vi "splitter.vi"(3 "Npp_Frame":i32, 4 "Current":dbl[](array[numeric]), 5 "Voltage":dbl[](array[numeric])) -> (1 "Current Array":dbl[][](array[numeric]), 2 "Voltage Array":dbl[][](array[numeric]))   [LabVIEW 2018]
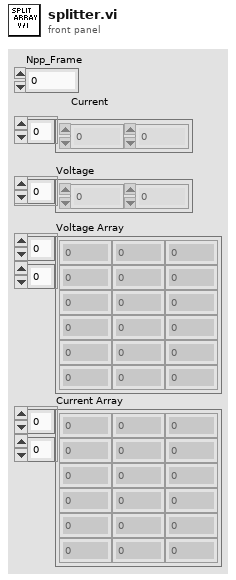
[diagram p1: front panel]
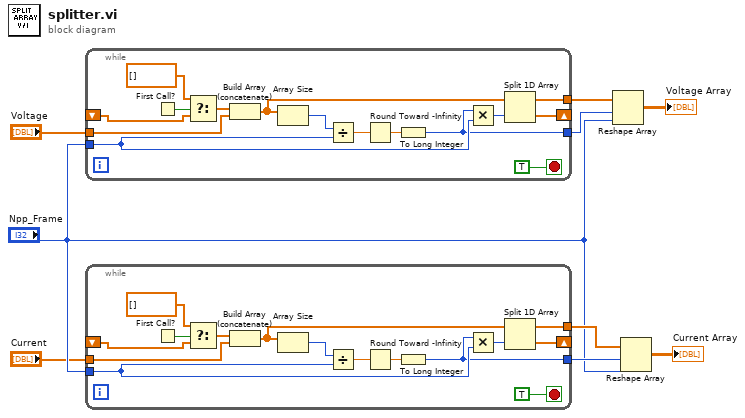
[diagram p0: block diagram]
diagram:
  n1 = while {
    tunnel: "Voltage" -> [w22]
    tunnel: [w24] -> w8
    shift-right: [w23] -> _
    shift-left: _ -> [w14]
    tunnel: "Npp_Frame" -> [w18]
    tunnel: [w11] -> w9
    stop <- TRUE stop-if-true
    n2 = First Call?() -> (First Call?: T/F=w15:bool)
    n3 = Select(t=dbl[] [], s=w15, f=w14) -> (s? t:f=w12:dbl[])
    n4 = Build Array (concatenate)(w12, w22) -> (w16:dbl[])
    n5 = Array Size(array=w16) -> (size(s)=w21:i32)
    n6 = Divide(x=w21, y=w18) -> (x/y=w20:dbl)
    n7 = Round Toward -Infinity(1:w20) -> (0:w19:dbl)
    n8 = To Long Integer(number=w19) -> (32bit integer=w11:i32)
    n9 = Multiply(x=w11, y=w18) -> (x*y=w17:i32)
    n10 = Split 1D Array(array=w16, index=w17) -> (first subarray=w24:dbl[], second subarray=w23:dbl[])
  }
  n11 = while {
    tunnel: "Current" -> [w37]
    tunnel: [w39] -> w4
    shift-right: [w38] -> _
    shift-left: _ -> [w29]
    tunnel: "Npp_Frame" -> [w33]
    tunnel: [w26] -> w5
    stop <- TRUE stop-if-true
    n12 = First Call?() -> (First Call?: T/F=w30:bool)
    n13 = Select(t=dbl[] [], s=w30, f=w29) -> (s? t:f=w27:dbl[])
    n14 = Build Array (concatenate)(w27, w37) -> (w31:dbl[])
    n15 = Array Size(array=w31) -> (size(s)=w36:i32)
    n16 = Divide(x=w36, y=w33) -> (x/y=w35:dbl)
    n17 = Round Toward -Infinity(1:w35) -> (0:w34:dbl)
    n18 = To Long Integer(number=w34) -> (32bit integer=w26:i32)
    n19 = Multiply(x=w26, y=w33) -> (x*y=w32:i32)
    n20 = Split 1D Array(array=w31, index=w32) -> (first subarray=w39:dbl[], second subarray=w38:dbl[])
  }
  n21 = Reshape Array(w8, w9, "Npp_Frame") -> (→"Voltage Array":dbl[][])
  n22 = Reshape Array(w4, w5, "Npp_Frame") -> (→"Current Array":dbl[][])
